vi "数据查询_仪器日志.vi"() -> ()   [LabVIEW 2016]
uses:
  <vilib>/Utility/miscctls.llb/LVRowAndColumnUnsignedTypeDef.ctl
  <vilib>/Utility/miscctls.llb/LVPointTypeDef.ctl
  <userlib>/_OpenG.lib/array/array.llb/Sort 2D Array (String)__ogtk.vi
panel:
  in  "导出":bool
  in  "查询":bool
  out "数据表":string[][](table)
  in  "结束日期":string="2020/01/01"
  in  "起始日期":string="2010/01/01"
  in  "组合框":string(combo)
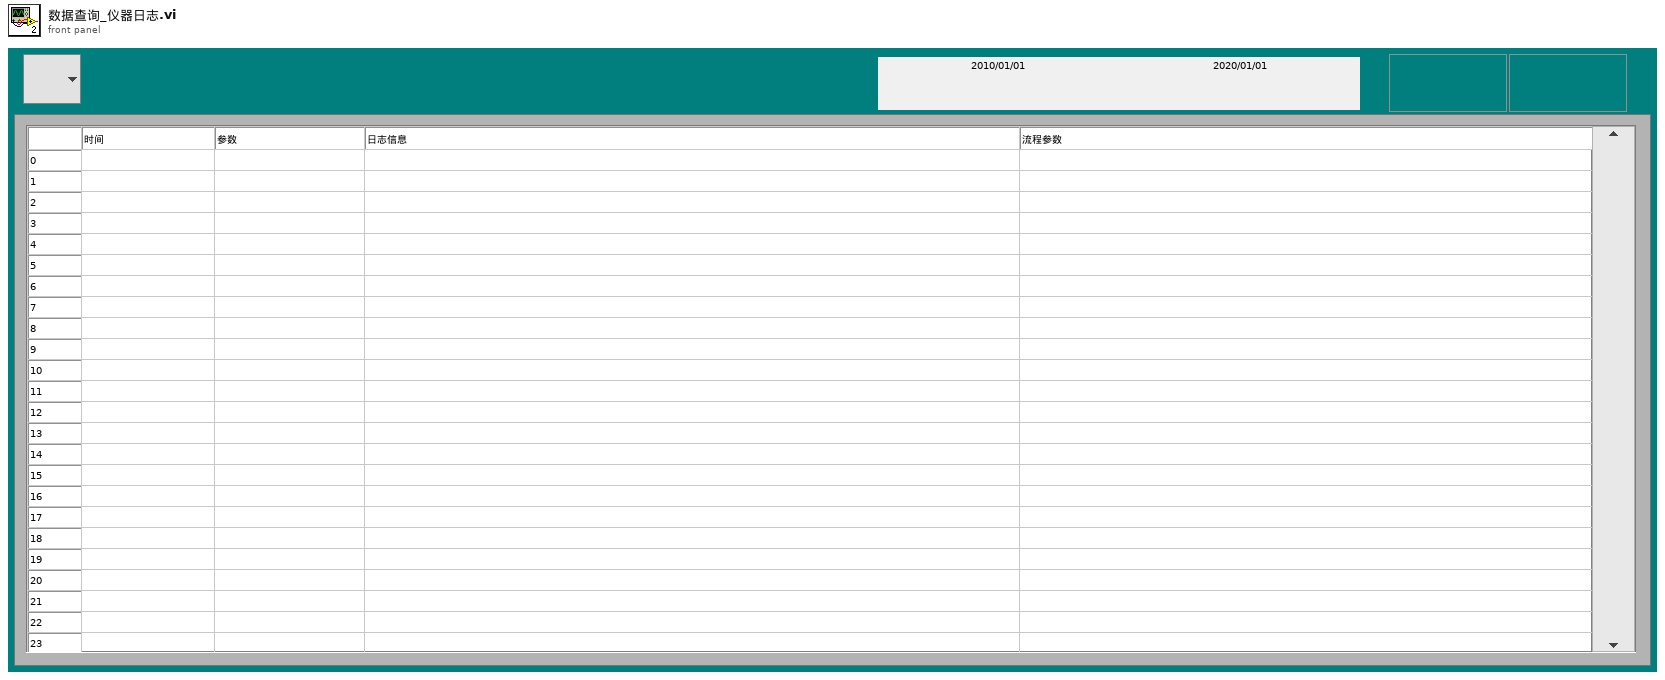
[diagram p1: front panel]
types:
  T1 = enum8{"Enabled", "Disabled", "Disabled and Grayed Out"}
  T2 = typedef "LVRowAndColumnUnsignedTypeDef.ctl" = cluster{"Row":u32, "Column":u32}
  T3 = typedef "LVPointTypeDef.ctl" = cluster{"Horizontal":i16, "Vertical":i16}
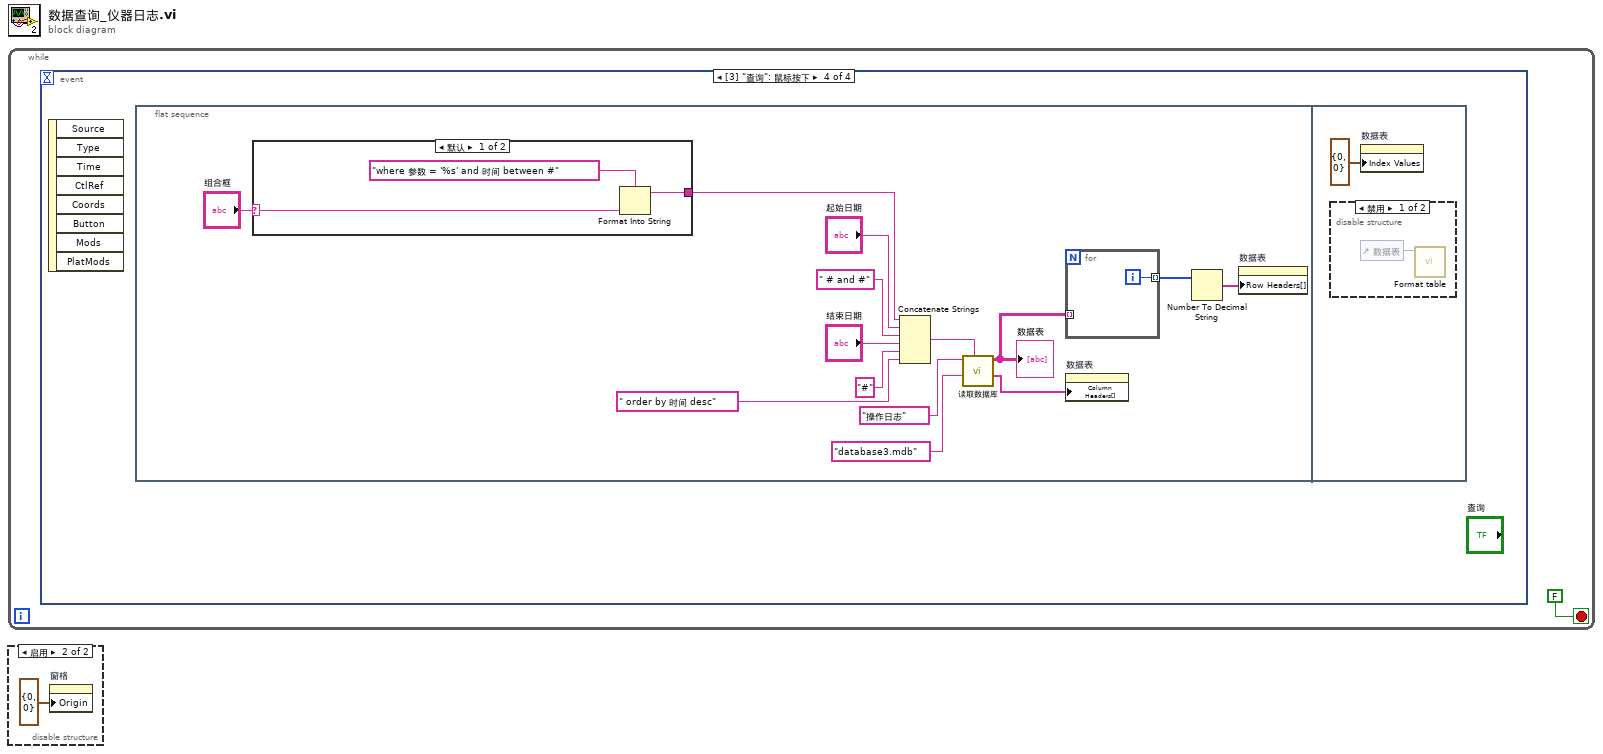
[diagram p0: block diagram]
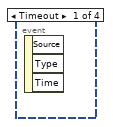
[diagram p2: hidden frame]
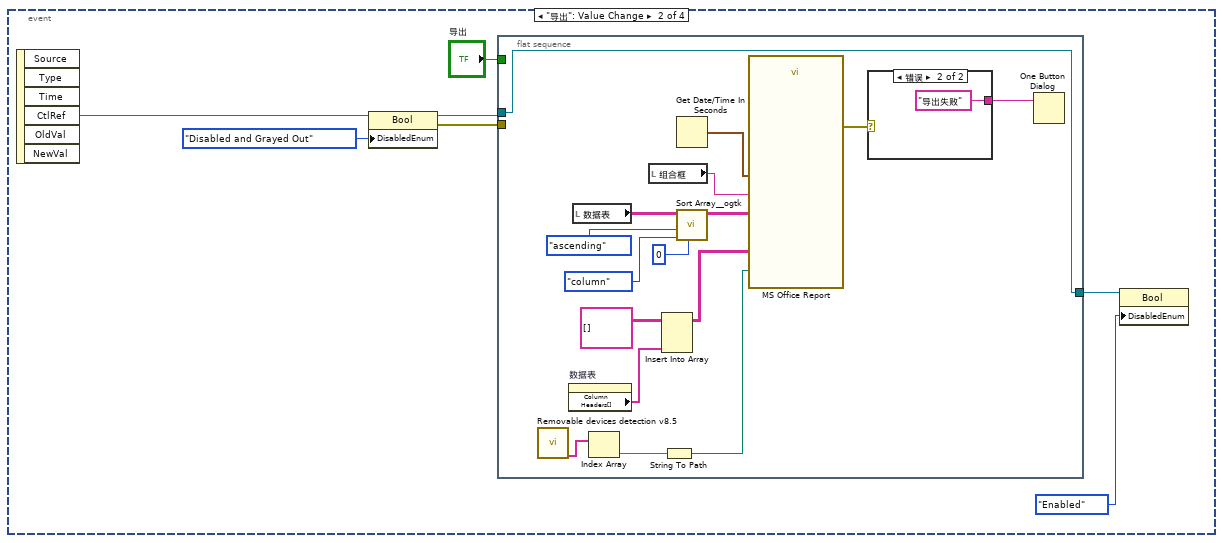
[diagram p3: hidden frame]
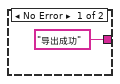
[diagram p4: hidden frame]
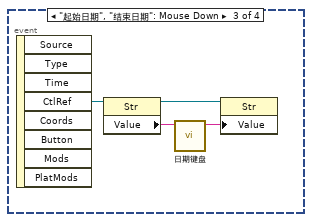
[diagram p5: hidden frame]
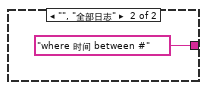
[diagram p6: hidden frame]
diagram:
  n1 = while {
    stop <- FALSE stop-if-true
    n2 = event shown="[3] \"查询\": 鼠标按下" {
      selector: _ -> [_ _ _ _]
      dyn-events: _ -> [_ _ _ _]
      timeout: _ -> [_ _ _ _]
      event Timeout {
        n3 = event-data() -> ()  [unwired: 1 in, 3 out]
      }
      event "导出": Value Change {
        n4 = event-data() -> ("CtlRef"=w2:refnum<vi>)  [unwired: 1 in, 5 out]
        n5 = property class="Bool"(reference=w2, "DisabledEnum"=T1."Disabled and Grayed Out" ("禁用")) -> (reference out=w6:refnum<vi>, error out=w7:errorcluster)  [unwired: 1 in]
        n6 = flat-sequence {
          tunnel: w7 -> [_]
          tunnel: [w17] -> w5
          tunnel: w6 -> [w17]
          tunnel: "导出" -> [_]
          frame #0 {
            n7 = call "Removable devices detection v8.5.vi"() -> ("Removable"=w14:string[])  [unwired: 4 out]
            n8 = property on="数据表" class="Tbl (严格)"() -> ("Column Headers[]"=w9:string[])  [unwired: 2 in, 2 out]
            n9 = local read "数据表"() -> (w23:string[][])
            n10 = Index Array(array=w14) -> (element=w13:string)  [unwired: 1 in]
            n11 = local read "组合框"() -> (w18:string)
            n12 = Insert Into Array(array=string[][] [], new element=w9) -> (w10:string[][])  [unwired: 2 in]
            n13 = String To Path(string=w13) -> (path=w12:path)
            n14 = Get Date/Time In Seconds() -> (seconds since 1Jan1904=w24:timestamp)
            n15 = call-poly <userlib>:"Sort Array__ogtk.vi"("Column/Row to Sort By"=u32 0, "Sort By in"=enum16{"row", "column"}."column", "Order"=enum16{"ascending", "descending"}."ascending", "Array in"=w23) -> ("Sorted Array out"=w22:string[][])  [unwired: 4 in, 3 out]
            n16 = call "MS Office Report"("Path to Save Report"=w12, "导出日期"=w24, "监测参数"=w18, "数据输入"=w22, "字段定义"=w10) -> ("error out"=w16:errorcluster)  [unwired: 21 in, 1 out]
            n17 = case shown="错误" w16 {
              tunnel: ["导出成功" ("消息") "导出失败" ("消息")] -> w15
              frame No Error {
              }
              frame Error {
              }
            }
            n18 = One Button Dialog(message=w15) -> ()  [unwired: 1 in, 1 out]
          }
        }
        n19 = property class="Bool"(reference=w5, "DisabledEnum"=T1."Enabled" ("禁用")) -> ()  [unwired: 1 in, 2 out]
      }
      event "起始日期", "结束日期": Mouse Down {
        n20 = event-data() -> ("CtlRef"=w30:refnum<vi>)  [unwired: 1 in, 7 out]
        n21 = property class="Str"(reference=w30) -> (reference out=w28:refnum<vi>, "Value"=w29:string)  [unwired: 1 in, 1 out]
        n22 = call "日期键盘.vi"("原值"=w29) -> ("x+y"=w27:string)  [unwired: 10 in]
        n23 = property class="Str"(reference=w28, "Value"=w27) -> ()  [unwired: 1 in, 2 out]
      }
      event "查询": Mouse Down {
        n24 = event-data() -> ()  [unwired: 1 in, 8 out]
        n25 = flat-sequence {
          frame #0 {
            n26 = case shown="默认" "组合框" {
              selector: "组合框" -> [w45 _]
              tunnel: [w47 "where 时间 between #" ("condition")] -> w31
              frame Default {
                n27 = Format Into String(format string="where 参数 = '%s' and 时间 between #" ("condition"), w45) -> (resulting string=w47:string)  [unwired: 2 in, 1 out]
              }
              frame "", "全部日志" {
              }
            }
            n28 = Concatenate Strings(w31, "起始日期", " # and #" ("condition"), "结束日期", "#" ("condition"), " order by 时间 desc" ("字符串")) -> (w43:string)
            n29 = call "读取数据库.vi"("condition"=w43, "database"="database3.mdb", "组合框"="操作日志") -> ("columns"=w39:string[], "表格"=w36:string[][])  [unwired: 5 in, 2 out]
            "数据表" <- w36
            n30 = for {
              tunnel: w36 -> [_] mode=indexing
              tunnel: [w49] -> w35 mode=indexing
              i -> [w49]
            }
            n31 = property on="数据表" class="Tbl (严格)"("Column Headers[]"=w39) -> ()  [unwired: 2 in, 2 out]
            n32 = Number To Decimal String(number=w35) -> (decimal integer string=w34:string[])  [unwired: 1 in]
            n33 = property on="数据表" class="Tbl (严格)"("Row Headers[]"=w34) -> ()  [unwired: 2 in, 2 out]
          }
          frame #1 {
            n34 = disable-structure shown="禁用" {
              frame Disabled {
                n35 = control-ref of="数据表"() -> (w51:refnum<vi>)
                n36 = call "Format table.vi"("Table输入"=w51) -> ()  [unwired: 11 in]
              }
              frame Enabled {
              }
            }
            n37 = property on="数据表" class="Tbl (严格)"("Index Values"=T2 {"Row"=0, "Column"=0} ("索引值")) -> ()  [unwired: 2 in, 2 out]
          }
        }
      }
    }
  }
  n38 = disable-structure shown="启用" {
    frame Disabled {
    }
    frame Enabled {
      n39 = property on="窗格" class="Pane"("Origin"=T3 {"Horizontal"=0, "Vertical"=0} ("原点")) -> ()  [unwired: 2 in, 2 out]
    }
  }
